vi "camTake.vi"() -> ()   [LabVIEW 2018]
uses:
  <vilib>/userdefined/High Color/IMAQdx.ctl
  <vilib>/vision/driver/NI_Vision_Acquisition_Software.lvlib
  <resource>/objmgr/imaqdx.rc
  <vilib>/vision/NI_Vision_Development_Module.lvlib
panel:
  in  "Numeric":i32
  out "P Image":T1(plugin-control) caption="Image Out"
  out "Found Objects":dbl[][](array[numeric]) format="%.2f"
  in  "Tab Control":T2(tab)
  in  "Hue B":cluster{"Lower value":i32, "Upper value":i32}={"Lower value"=80, "Upper value"=241}
  in  "Saturation B":cluster{"Lower value":i32, "Upper value":i32}={"Lower value"=37, "Upper value"=255}
  in  "Luma B":cluster{"Lower value":i32, "Upper value":i32}={"Lower value"=62, "Upper value"=255}
  in  "Luma R":cluster{"Lower value":i32, "Upper value":i32}={"Lower value"=0, "Upper value"=255}
  in  "Hue R":cluster{"Lower value":i32, "Upper value":i32}={"Lower value"=0, "Upper value"=255}
  in  "Saturation R":cluster{"Lower value":i32, "Upper value":i32}={"Lower value"=0, "Upper value"=255}
  in  "Hue O":cluster{"Lower value":i32, "Upper value":i32}={"Lower value"=0, "Upper value"=255}
  in  "Saturation O":cluster{"Lower value":i32, "Upper value":i32}={"Lower value"=0, "Upper value"=255}
  in  "Luma O":cluster{"Lower value":i32, "Upper value":i32}={"Lower value"=0, "Upper value"=255}
  in  "Hue G":cluster{"Lower value":i32, "Upper value":i32}={"Lower value"=0, "Upper value"=255}
  in  "Saturation G":cluster{"Lower value":i32, "Upper value":i32}={"Lower value"=0, "Upper value"=255}
  in  "Luma G":cluster{"Lower value":i32, "Upper value":i32}={"Lower value"=0, "Upper value"=255}
  in  "Hue Y":cluster{"Lower value":i32, "Upper value":i32}={"Lower value"=0, "Upper value"=255}
  in  "Saturation Y":cluster{"Lower value":i32, "Upper value":i32}={"Lower value"=0, "Upper value"=255}
  in  "Luma Y":cluster{"Lower value":i32, "Upper value":i32}={"Lower value"=0, "Upper value"=255}
  in  "color":string
  in  "stop":bool
  out "Image Out":T1(plugin-control)
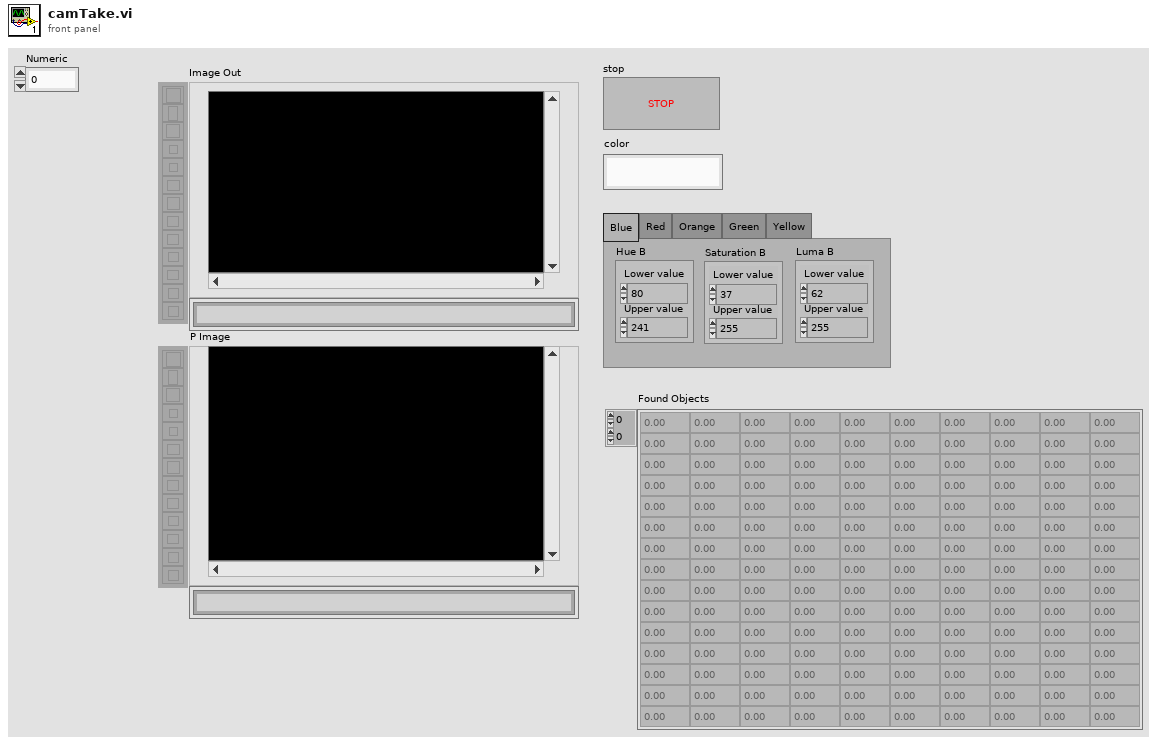
[diagram p1: front panel]
types:
  T1 = typedef "IMAQ Image.ctl" = refnum<image>
  T2 = enum32{"Blue", "Red", "Orange", "Green", "Yellow"}
  T3 = typedef "IMAQdx.ctl" = refnum<k21>
  T4 = typedef "Particle Parameters" = i32
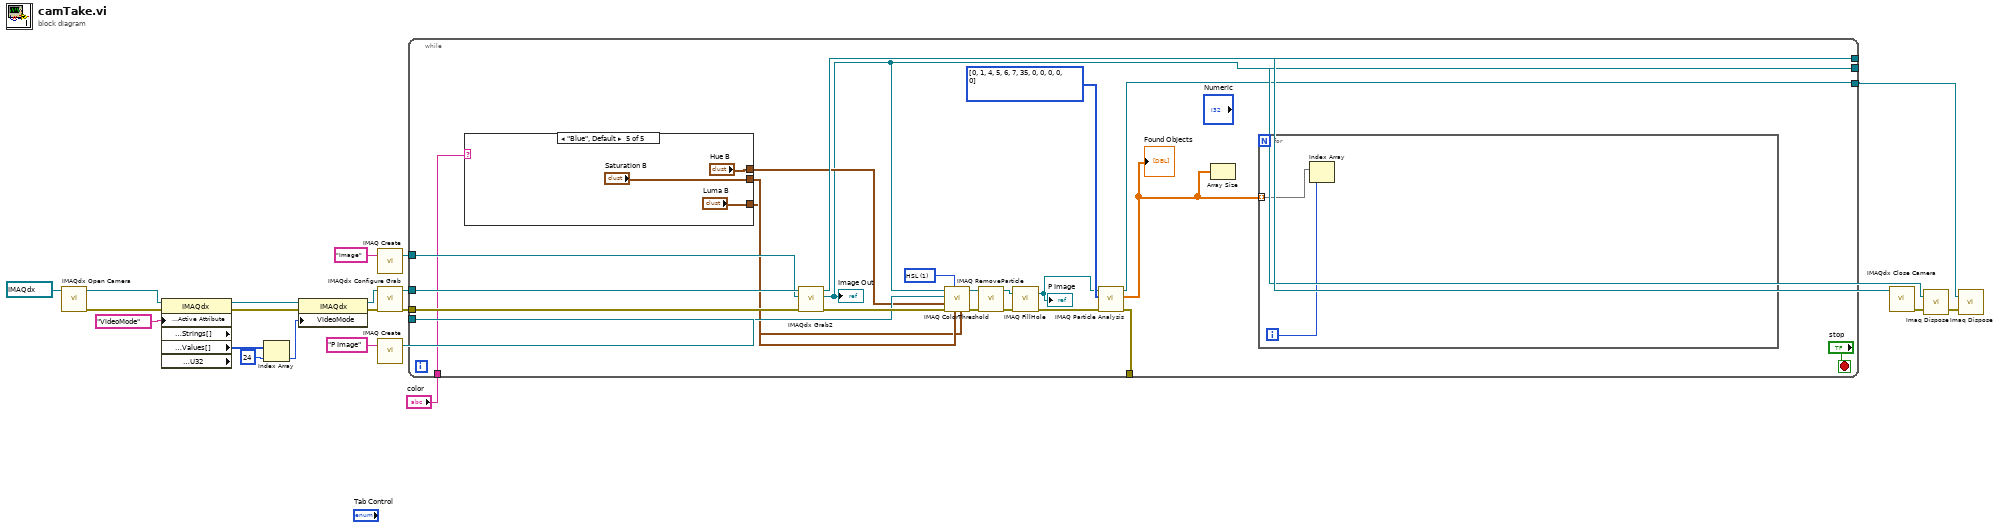
[diagram p0: block diagram]
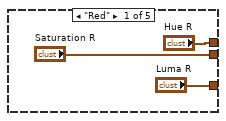
[diagram p2: hidden frame]
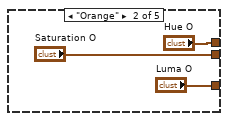
[diagram p3: hidden frame]
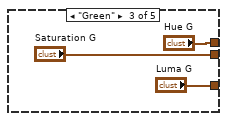
[diagram p4: hidden frame]
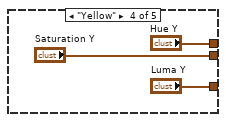
[diagram p5: hidden frame]
diagram:
  n1 = call <vilib>:"IMAQdx Open Camera.vi"("Session In"=T3 "cam1") -> ("error out"=w20:errorcluster, "Session Out"=w21:T3)  [unwired: 9 in]
  n2 = property class="IMAQdx" props=["Camera Attributes:Active Attribute", "Camera Attributes:Enum:Strings[]", "Camera Attributes:Enum:Values[]", "Camera Attributes:Value:U32"](reference=w21, error in=w20, "Camera Attributes:Active Attribute"="VideoMode" ("ActiveAttribute")) -> (reference out=w16:T3, error out=w15:errorcluster, "Camera Attributes:Enum:Values[]"=w19:u32[])  [unwired: 2 out]
  n3 = Index Array(array=w19, index=24) -> (element=w17:u32)
  n4 = property class="IMAQdx"(reference=w16, error in=w15, "VideoMode"=w17) -> (reference out=w13:T3, error out=w14:errorcluster)
  n5 = call "IMAQ Create"("Image Name"="Image") -> ("New Image"=w9:T1)  [unwired: 4 in, 1 out]
  n6 = call <vilib>:"IMAQdx Configure Grab.vi"("error in"=w14, "Session In"=w13) -> ("error out"=w11:errorcluster, "Session Out"=w12:T3)  [unwired: 8 in]
  n7 = call "IMAQ Create"("Image Name"="P Image") -> ("New Image"=w3:T1)  [unwired: 4 in, 1 out]
  n8 = while {
    tunnel: w9 -> [w44]
    tunnel: w12 -> [w46]
    tunnel: [w43] -> w8
    tunnel: w11 -> [w45]
    tunnel: [w24] -> w6
    tunnel: w3 -> [w40]
    tunnel: [w31] -> w2
    tunnel: "color" -> [w30]
    tunnel: [w25] -> _
    stop <- "stop" stop-if-true
    w33 = T4[] [0, 1, 4, 5, 6, 7, 35, 0, 0, 0, 0, 0] items=["Center of Mass X", "Center of Mass Y", "First Pixel X", "First Pixel Y", "Bounding Rect Left", "Bounding Rect Top", "Bounding Rect Right", "Bounding Rect Bottom", "Max Feret Diameter Start X", "Max Feret Diameter Start Y", "Max Feret Diameter End X", "Max Feret Diameter End Y", "Max Horiz. Segment Length Left", "Max Horiz. Segment Length Right", "Max Horiz. Segment Length Row", "-", "Bounding Rect Width", "Bounding Rect Height", "Bounding Rect Diagonal", "Perimeter", "Convex Hull Perimeter", "Holes' Perimeter", "Max Feret Diameter", "Equivalent Ellipse Major Axis", "Equivalent Ellipse Minor Axis", "Equivalent Ellipse Minor Axis (Feret)", "Equivalent Rect Long Side", "Equivalent Rect Short Side", "Equivalent Rect Diagonal", "Equivalent Rect Short Side (Feret)", "Average Horiz. Segment Length", "Average Vert. Segment Length", "Hydraulic Radius", "Waddel Disk Diameter", "-", "Area", "Holes' Area", "Particle & Holes' Area", "Convex Hull Area", "Image Area", "-", "Number of Holes", "Number of Horiz. Segments", "Number of Vert. Segments", "-", "Orientation", "Max Feret Diameter Orientation", "-", "% Area/Image Area", "% Area/(Particle & Holes' Area)", "Ratio of Equivalent Ellipse Axes", "Ratio of Equivalent Rect Sides", "-", "Elongation Factor", "Compactness Factor", "Heywood Circularity Factor", "Type Factor", "-", "Sum X", "Sum Y", "Sum XX", "Sum XY", "Sum YY", "Sum XXX", "Sum XXY", "Sum XYY", "Sum YYY", "-", "Moment of Inertia XX", "Moment of Inertia XY", "Moment of Inertia YY", "Moment of Inertia XXX", "Moment of Inertia XXY", "Moment of Inertia XYY", "Moment of Inertia YYY", "Norm. Moment of Inertia XX", "Norm. Moment of Inertia XY", "Norm. Moment of Inertia YY", "Norm. Moment of Inertia XXX", "Norm. Moment of Inertia XXY", "Norm. Moment of Inertia XYY", "Norm. Moment of Inertia YYY", "Hu Moment 1", "Hu Moment 2", "Hu Moment 3", "Hu Moment 4", "Hu Moment 5", "Hu Moment 6", "Hu Moment 7"] ("Pixel Measurements")
    w39 = u16 1 items=["RGB", "HSL", "HSV", "HSI"] ("Color Mode")
    n9 = case shown="\"Blue\", Default" w30 {
      tunnel: ["Hue R" "Hue O" "Hue G" "Hue Y" "Hue B"] -> w29
      tunnel: ["Saturation R" "Saturation O" "Saturation G" "Saturation Y" "Saturation B"] -> w28
      tunnel: ["Luma R" "Luma O" "Luma G" "Luma Y" "Luma B"] -> w27
      frame "Red" {
      }
      frame "Orange" {
      }
      frame "Green" {
      }
      frame "Yellow" {
      }
      frame "Blue", Default {
      }
    }
    n10 = call <vilib>:"IMAQdx Grab2.vi"("error in"=w45, "Image In"=w44, "Session In"=w46) -> ("error out"=w41:errorcluster, "Image Out"=w24:T1, "Session Out"=w43:T3)  [unwired: 5 in, 1 out]
    "Image Out" <- w24
    n11 = call "IMAQ ColorThreshold"("Blue or Luma or Val or Inten Range"=w27, "Green or Sat Range"=w28, "Color Mode"=w39, "error in (no error)"=w41, "Red or Hue Range"=w29, "Image Dst"=w40, "Image Src"=w24) -> ("error out"=w38:errorcluster, "Image Dst Out"=w37:T1)  [unwired: 3 in]
    n12 = call "IMAQ RemoveParticle"("error in (no error)"=w38, "Image Src"=w37) -> ("error out"=w36:errorcluster, "Image Dst Out"=w35:T1)  [unwired: 8 in]
    n13 = call "IMAQ FillHole"("error in (no error)"=w36, "Image Src"=w35) -> ("error out"=w34:errorcluster, "Image Dst Out"=w32:T1)  [unwired: 4 in]
    "P Image" <- w32
    n14 = call "IMAQ Particle Analysis"("error in (no error)"=w34, "Pixel Measurements"=w33, "Image"=w32) -> ("error out"=w25:errorcluster, "Particle Measurements (Pixels)"=w26:dbl[][], "Image Out (duplicate)"=w31:T1)  [unwired: 3 in, 3 out]
    "Found Objects" <- w26
    n15 = Array Size(array=w26) -> ()  [unwired: 1 out]
    n16 = for {
      tunnel: w26 -> [w48] mode=indexing
      i -> [w47]
      n17 = Index Array(array=w48, index=w47) -> ()  [unwired: 1 out]
    }
  }
  n18 = call <vilib>:"IMAQdx Close Camera.vi"("Session In"=w8) -> ("error out"=w7:errorcluster)  [unwired: 10 in]
  n19 = call "Imaq Dispose"("Image"=w6, "error in (no error)"=w7) -> ("error out"=w4:errorcluster)  [unwired: 4 in]
  n20 = call "Imaq Dispose"("Image"=w2, "error in (no error)"=w4) -> ()  [unwired: 4 in, 1 out]
